vi "Text Get Event Fragment.vi"(2 "Event":string[][](array[string]), 3 "Fragment Type":string) -> (0 "Fragment":string, 1 "Found":bool)   [LabVIEW 2019]
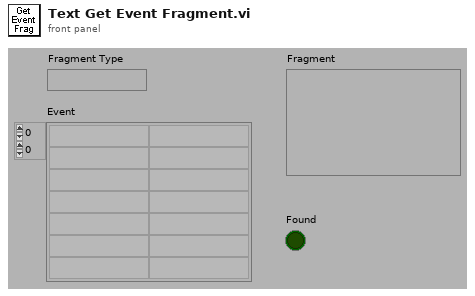
[diagram p1: front panel]
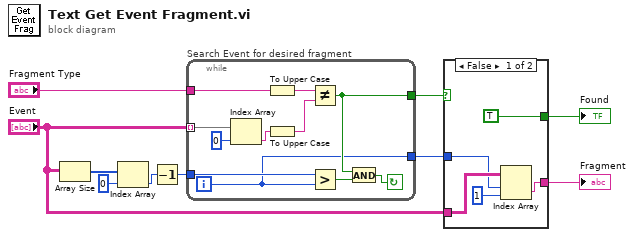
[diagram p0: block diagram]
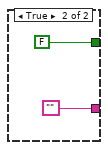
[diagram p2: hidden frame]
diagram:
  n1 = Array Size(array="Event") -> (size(s)=w9:i32[])
  n2 = Index Array(array=w9, index=0 ("Index")) -> (element=w7:i32)
  n3 = Decrement(x=w7) -> (x-1=w6:i32)
  n4 = while "Search Event for desired fragment" {
    tunnel: [w13] -> w5
    tunnel: [w11] -> w3
    tunnel: w6 -> [w12]
    tunnel: "Fragment Type" -> [w21]
    tunnel: "Event" -> [w16] mode=indexing
    i -> [w11]
    stop <- w14 continue-if-true
    n5 = Index Array(array=w16, index=0 ("Index")) -> (element=w19:string)
    n6 = To Upper Case(1:w21) -> (0:w17:string)
    n7 = To Upper Case(1:w19) -> (0:w18:string)
    n8 = Not Equal?(x=w17, y=w18) -> (x != y?=w13:bool)
    n9 = Greater?(x=w12, y=w11) -> (0:w15:bool)
    n10 = And(x=w13, y=w15) -> (x .and. y?=w14:bool)
  }
  n11 = case shown="False" w5 {
    tunnel: "Event" -> [w26 _]
    tunnel: w3 -> [w25 _]
    tunnel: [w23 ""] -> w2
    tunnel: [TRUE FALSE] -> w1
    frame False {
      n12 = Index Array(array=w26, index (row)=w25, index (col)=1 ("Index")) -> (element=w23:string)
    }
    frame True {
    }
  }
  "Fragment" <- w2
  "Found" <- w1
